vi "Swerve Drive.vi"(1 "Rot. Point Y":dbl, 3 "Rot. Point X":dbl) -> ()   [LabVIEW 2018]
uses:
  Robot Global Data.vi
  <vilib>/Rock Robotics/WPI/ThirdParty/Phoenix-LabVIEW/Motor Controller/Controls/CTRE_Phoenix_MotorControl_ControlMode.ctl
panel:
  # "SWERVE DRIVE\nVersion 3.1\n\nCory Lynch\nApple Pi Robotics\nTeam 2067"
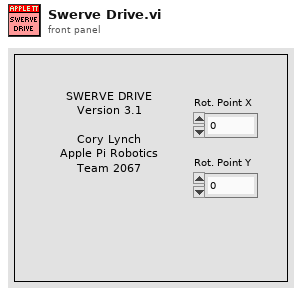
[diagram p1: front panel]
types:
  T1 = enum16{"Back Left", "Back Right", "Front Left", "Front Right"}
  T2 = typedef "CTRE_Phoenix_MotorControl_ControlMode.ctl" = u16
  T3 = typedef "WPI_MotorControlDeviceRef.ctl" = cluster{"DeviceStatus":errorcluster, "Type":T4, "PWM":cluster{"PWM Channel":T5, "DeadBand":T6}, "CAN":cluster{"Device Number":u8, "SetOutput VI Ref":variant, "GetOutput VI Ref":variant, "Enable VI Ref":variant, "Disable VI Ref":variant, "Data":variant}, "Invert":bool, "DIO PWM":cluster{"PWM \"Enable\" Channel":T5, "DIOChannel":T7, "PWM Rate":dbl}}
  T4 = typedef "WPI_MotorControlType.ctl" = enum16{"PWM", "CAN", "DIO PWM"}
  T5 = typedef "FPGA_DIOPWMChannel.ctl" = enum8{"PWM 0", "PWM 1", "PWM 2", "PWM 3", "PWM 4", "PWM 5", "PWM 6", "PWM 7", "PWM 8", "PWM 9", "PWM MXP 0", "PWM MXP 1", "PWM MXP 2", "PWM MXP 3", "PWM MXP 4", "PWM MXP 5", "PWM MXP 6", "PWM MXP 7", "PWM MXP 8", "PWM MXP 9", "Invalid"}
  T6 = typedef "WPI_PWMDeadband.ctl" = cluster{"Name":string, "maxPositivePwm":i32, "minPositivePwm":i32, "centerPwm":i32, "maxNegativePwm":i32, "minNegativePwm":i32, "angularRange":u16}
  T7 = typedef "FPGA_DIOChannel.ctl" = enum8{"DIO 0", "DIO 1", "DIO 2", "DIO 3", "DIO 4", "DIO 5", "DIO 6", "DIO 7", "DIO 8", "DIO 9", "DIO MXP 0", "DIO MXP 1", "DIO MXP 2", "DIO MXP 3", "DIO MXP 4", "DIO MXP 5", "DIO MXP 6", "DIO MXP 7", "DIO MXP 8", "DIO MXP 9", "DIO MXP 10", "DIO MXP 11", "DIO MXP 12", "DIO MXP 13", "DIO MXP 14", "DIO MXP 15", "SPI Port CS1", "SPI Port CS2", "SPI Port CS3", "SPI Port MISO", "SPI Port MOSI", "Invalid"}
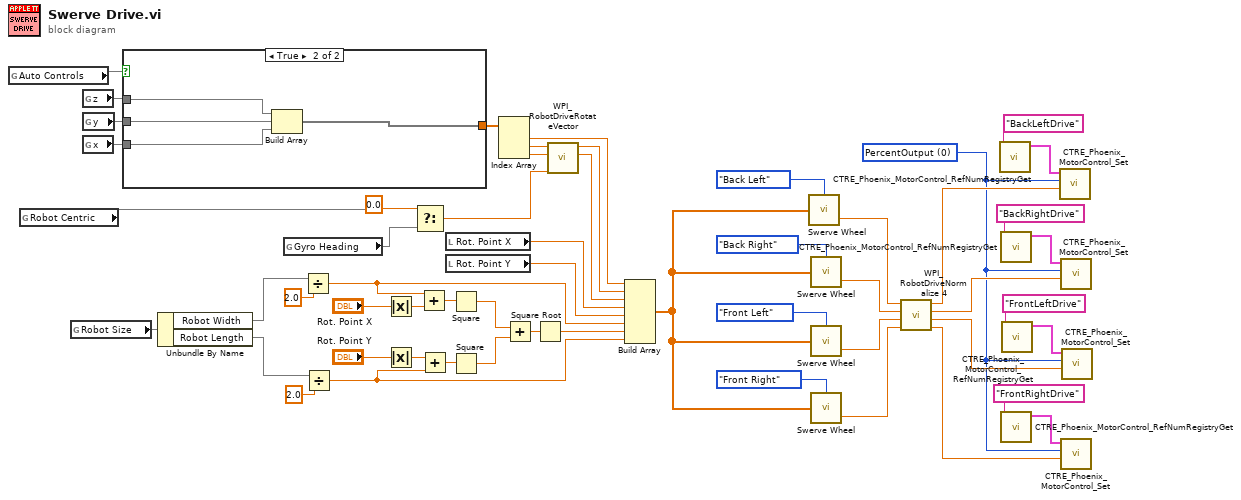
[diagram p0: block diagram]
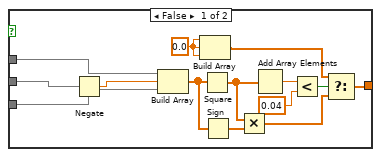
[diagram p2: hidden frame]
diagram:
  w10 = T2 0 items=["PercentOutput"=0, "Position"=1, "Velocity"=2, "Current"=3, "Follower"=5, "MotionProfile"=6, "MotionMagic"=7, "MotionProfileArc"=10, "Disabled"=15] ("Control Mode")
  n1 = global read "Robot Global Data.vi" "Auto Controls"() -> (w2)
  n2 = global read "Robot Global Data.vi" "Robot Centric"() -> (w3)
  n3 = global read "Robot Global Data.vi" "Robot Size"() -> (w9)
  n4 = global read "Robot Global Data.vi" "z"() -> (w12)
  n5 = global read "Robot Global Data.vi" "y"() -> (w11)
  n6 = global read "Robot Global Data.vi" "x"() -> (w13)
  n7 = case shown="True" w2 {
    tunnel: w11 -> [w58 w70]
    tunnel: w13 -> [w56 w73]
    tunnel: w12 -> [w59 w71]
    tunnel: [w61 w72] -> w20
    frame False {
      w65 = 0.0 ("element")
      n8 = Negate(x=w58) -> (-x=w57:dbl)
      n9 = Build Array(w59, w57, w56) -> (w60:dbl[])
      n10 = Build Array(w65, w65, w65) -> (w66:dbl[])
      n11 = Square(x=w60) -> (x^2=w63:dbl[])
      n12 = Sign(1:w60) -> (0:w64:dbl[])
      n13 = Multiply(x=w63, y=w64) -> (x*y=w62:dbl[])
      n14 = Add Array Elements(numeric array=w63) -> (sum=w69:dbl)
      n15 = Less?(x=w69, y=0.04 ("x")) -> (x < y?=w67:bool)
      n16 = Select(t=w66, s=w67, f=w62) -> (s? t:f=w61:dbl[])
    }
    frame True {
      n17 = Build Array(w71, w70, w73) -> (w72:void[])
    }
  }
  n18 = Unbundle By Name(w9) -> ("Robot Width"=w7, "Robot Length"=w8)
  n19 = global read "Robot Global Data.vi" "Gyro Heading"() -> (w1)
  n20 = Divide(x=w7, y=2.0) -> (x/y=w24:dbl)
  n21 = Divide(x=w8, y=2.0) -> (x/y=w22:dbl)
  n22 = Absolute Value(x="Rot. Point X") -> (abs(x)=w38:dbl)
  n23 = Absolute Value(x="Rot. Point Y") -> (abs(x)=w36:dbl)
  n24 = Select(t=0.0, s=w3, f=w1) -> (s? t:f=w16:dbl)
  n25 = Add(x=w24, y=w38) -> (x+y=w37:dbl)
  n26 = Add(x=w36, y=w22) -> (x+y=w35:dbl)
  n27 = local read "Rot. Point X"() -> (w26:dbl)
  n28 = local read "Rot. Point Y"() -> (w25:dbl)
  n29 = Square(x=w37) -> (x^2=w33:dbl)
  n30 = Square(x=w35) -> (x^2=w34:dbl)
  n31 = Index Array(array=w20) -> (element #1=w15:dbl, element #2=w21:dbl, element #3=w27:dbl)  [unwired: 3 in]
  n32 = Add(x=w33, y=w34) -> (x+y=w32:dbl)
  n33 = Square Root(x=w32) -> (sqrt(x)=w23:dbl)
  n34 = call <vilib>:"WPI_RobotDriveRotateVector.vi"("Angle"=w16, "X"=w27, "Y"=w21) -> ("X'"=w18:dbl, "Y'"=w14:dbl)  [unwired: 7 out]
  n35 = Build Array(w15, w14, w18, w26, w25, w24, w23, w22) -> (w19:dbl[])
  n36 = call "Swerve Wheel.vi"("Wheel"=T1."Back Left", "Inputs"=w19) -> ("Speed"=w55:dbl)  [unwired: 3 in]
  n37 = call "Swerve Wheel.vi"("Wheel"=T1."Back Right", "Inputs"=w19) -> ("Speed"=w54:dbl)  [unwired: 3 in]
  n38 = call "Swerve Wheel.vi"("Wheel"=T1."Front Left", "Inputs"=w19) -> ("Speed"=w53:dbl)  [unwired: 3 in]
  n39 = call "Swerve Wheel.vi"("Wheel"=T1."Front Right", "Inputs"=w19) -> ("Speed"=w52:dbl)  [unwired: 3 in]
  n40 = call <vilib>:"WPI_RobotDriveNormalize 4.vi"("D"=w52, "C"=w53, "B"=w54, "A"=w55) -> ("D'"=w39:dbl, "C'"=w40:dbl, "B'"=w41:dbl, "A'"=w42:dbl)
  n41 = call <vilib>:"CTRE_Phoenix_MotorControl_RefNumRegistryGet.vi"("refnum name"="BackLeftDrive") -> ("PhoenixMotorControlDevRef"=w50:T3)  [unwired: 9 in, 1 out]
  n42 = call <vilib>:"CTRE_Phoenix_MotorControl_RefNumRegistryGet.vi"("refnum name"="BackRightDrive") -> ("PhoenixMotorControlDevRef"=w47:T3)  [unwired: 9 in, 1 out]
  n43 = call <vilib>:"CTRE_Phoenix_MotorControl_RefNumRegistryGet.vi"("refnum name"="FrontRightDrive") -> ("PhoenixMotorControlDevRef"=w43:T3)  [unwired: 9 in, 1 out]
  n44 = call <vilib>:"CTRE_Phoenix_MotorControl_RefNumRegistryGet.vi"("refnum name"="FrontLeftDrive") -> ("PhoenixMotorControlDevRef"=w46:T3)  [unwired: 9 in, 1 out]
  n45 = call <vilib>:"CTRE_Phoenix_MotorControl_Set.vi"("Output"=w42, "Control Mode"=w10, "PhoenixMotorControlDevRef"=w50) -> ()  [unwired: 7 in, 2 out]
  n46 = call <vilib>:"CTRE_Phoenix_MotorControl_Set.vi"("Output"=w41, "Control Mode"=w10, "PhoenixMotorControlDevRef"=w47) -> ()  [unwired: 7 in, 2 out]
  n47 = call <vilib>:"CTRE_Phoenix_MotorControl_Set.vi"("Output"=w39, "Control Mode"=w10, "PhoenixMotorControlDevRef"=w43) -> ()  [unwired: 7 in, 2 out]
  n48 = call <vilib>:"CTRE_Phoenix_MotorControl_Set.vi"("Output"=w40, "Control Mode"=w10, "PhoenixMotorControlDevRef"=w46) -> ()  [unwired: 7 in, 2 out]
